vi "Setup Statically-Linked subWorkers.vi"(8 "error in":errorcluster, 11 "Manager Panel in":refnum<class "Manager Panel.lvclass">) -> (0 "error out":errorcluster, 3 "Manager Panel out":refnum<class "Manager Panel.lvclass">)   [LabVIEW 2020, in "Manager Panel.lvclass"]
doc: "This VI performs a setup of all the statically-linked subWorkers that belong to the Worker that owns this VI. This VI must be called <b>before</b> any statically-linked subWorkers are called."
uses:
  Manager Panel.lvclass
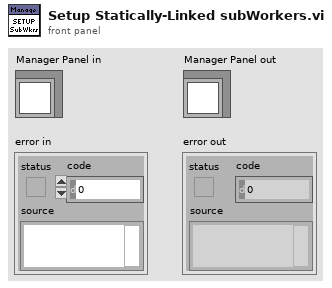
[diagram p1: front panel]
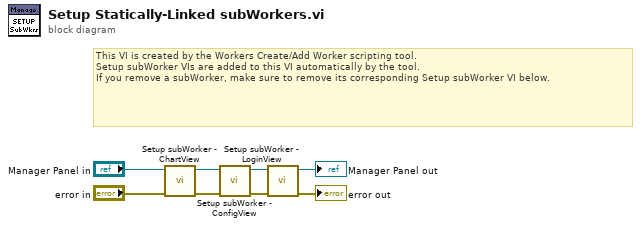
[diagram p0: block diagram]
diagram:
  # "This VI is created by the Workers Create/Add Worker scripting tool.\nSetup subWorker VIs are added to this VI automatically by the tool.\nIf you remove a subWorker, make sure to remove its corresponding Setup subWorker VI below."
  n1 = call "Setup subWorker - ChartView.vi"("error in"="error in", "Manager Panel in"="Manager Panel in") -> ("error out"=w7:errorcluster, "Manager Panel out"=w4:refnum<class "Manager Panel.lvclass">)  [unwired: 8 in]
  n2 = call "Setup subWorker - ConfigView.vi"("error in"=w7, "Manager Panel in"=w4) -> ("error out"=w5:errorcluster, "Manager Panel out"=w2:refnum<class "Manager Panel.lvclass">)  [unwired: 8 in]
  n3 = call "Setup subWorker - LoginView.vi"("error in"=w5, "Manager Panel in"=w2) -> ("error out"=→"error out":errorcluster, "Manager Panel out"=→"Manager Panel out":refnum<class "Manager Panel.lvclass">)  [unwired: 8 in]
